vi "HTML Block Diagram Save.vi"(5 "url":string, 7 "title":string="bd.html", 8 "error in":errorcluster, 9 "sub vi loc":T1[](array[typedef]), 10 "sub vi refs":refnum<vi>[](array[refnum]), 11 "base path":path) -> (0 "error out":errorcluster)   [LabVIEW 2014, in "lvprj2html.lvlib"]
uses:
  lvprj2html.lvlib
  <vilib>/Utility/miscctls.llb/LVRectTypeDef.ctl
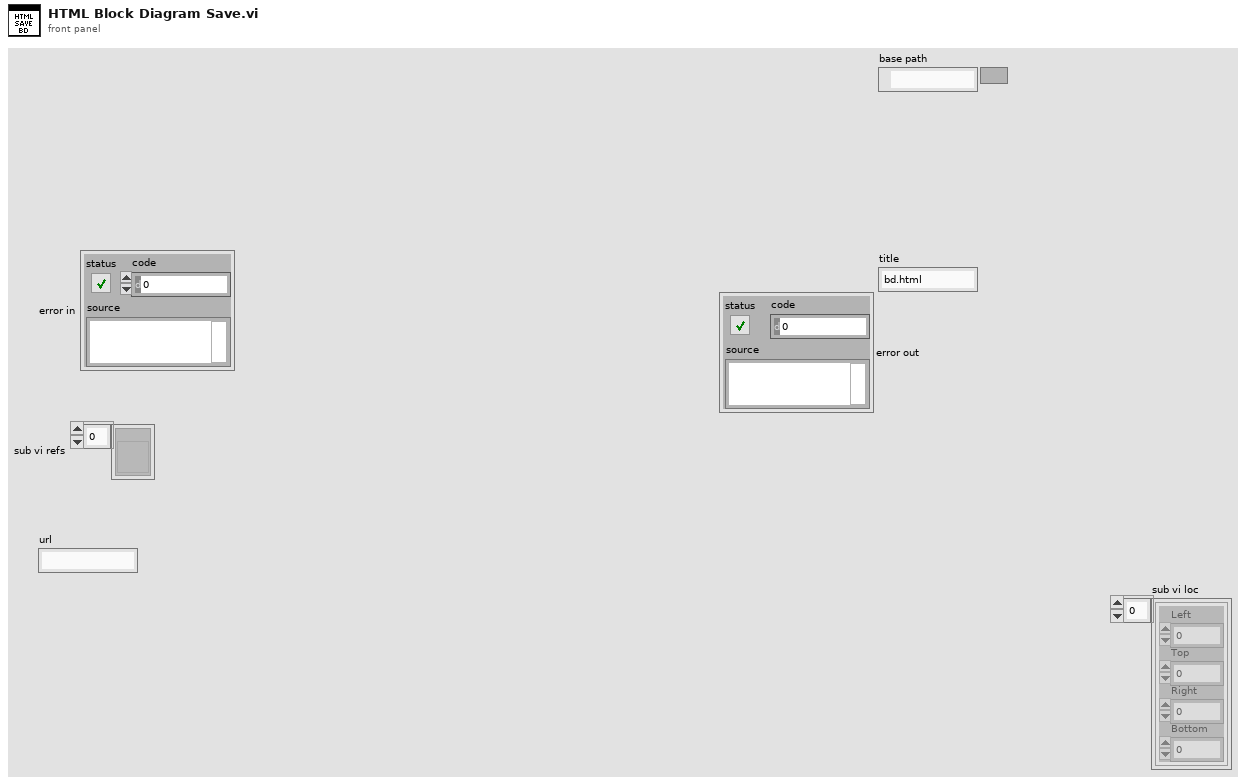
[diagram p1: front panel]
types:
  T1 = typedef "LVRectTypeDef.ctl" = cluster{"Left":i16, "Top":i16, "Right":i16, "Bottom":i16}
  T2 = enum16{"open", "replace", "create", "open or create", "replace or create", "replace or create with confirmation"}
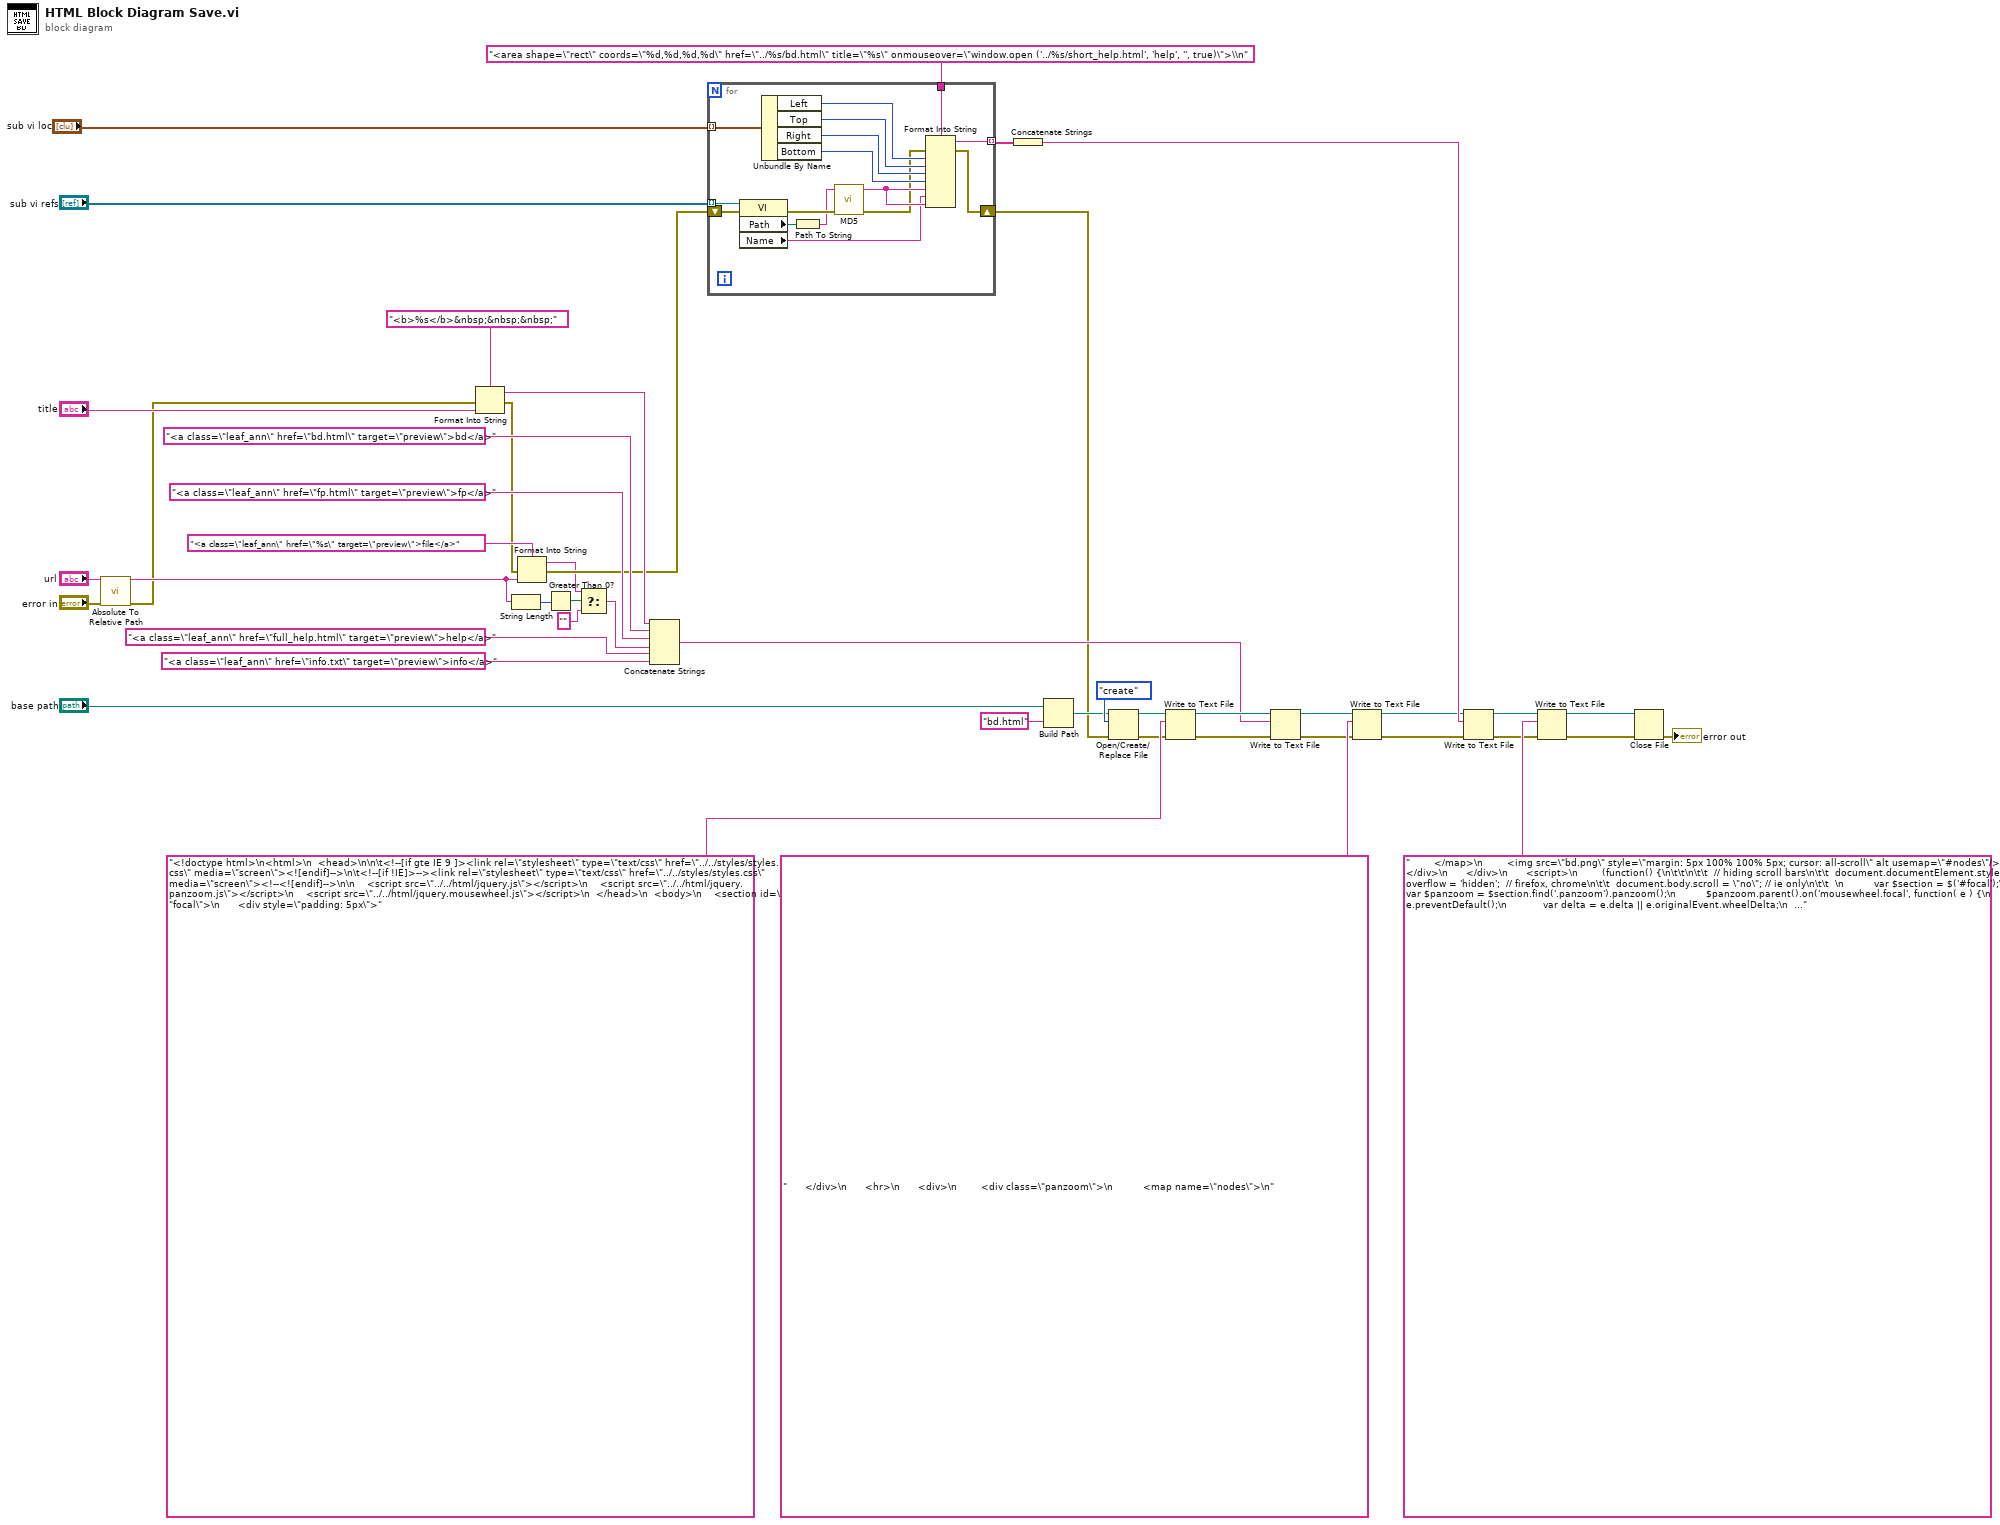
[diagram p0: block diagram]
diagram:
  n1 = call "Absolute To Relative Path.vi"("url in"="url", "error in (no error)"="error in") -> ("url out"=w4:string, "error out"=w3:errorcluster)  [unwired: 12 in]
  n2 = Format Into String(format string="<b>%s</b>&nbsp;&nbsp;&nbsp;", error in=w3, "title") -> (resulting string=w34:string, error out=w13:errorcluster)  [unwired: 1 in]
  n3 = String Length(string=w4) -> (length=w10:i32)
  n4 = Format Into String(format string="<a class=\"leaf_ann\" href=\"%s\" target=\"preview\">file</a>" ("text"), error in=w13, w4) -> (resulting string=w7:string, error out=w12:errorcluster)  [unwired: 1 in]
  n5 = Greater Than 0?(x=w10) -> (x > 0?=w9:bool)
  n6 = Select(t=w7, s=w9, f="") -> (s? t:f=w6:string)
  n7 = Concatenate Strings(w34, "<a class=\"leaf_ann\" href=\"bd.html\" target=\"preview\">bd</a>" ("text"), "<a class=\"leaf_ann\" href=\"fp.html\" target=\"preview\">fp</a>" ("text"), w6, "<a class=\"leaf_ann\" href=\"full_help.html\" target=\"preview\">help</a>" ("text"), "<a class=\"leaf_ann\" href=\"info.txt\" target=\"preview\">info</a>" ("text")) -> (w24:string)
  n8 = for {
    tunnel: "<area shape=\"rect\" coords=\"%d,%d,%d,%d\" href=\"../%s/bd.html\" title=\"%s\" onmouseover=\"window.open ('../%s/short_help.html', 'help', '', true)\">\\n" ("format string") -> [w62]
    tunnel: "sub vi loc" -> [w61] mode=indexing
    tunnel: [w56] -> w39 mode=indexing
    shift-right: [w54] -> w11
    shift-left: w12 -> [w51]
    tunnel: "sub vi refs" -> [w52] mode=indexing
    n9 = property class="VI"(reference=w52, error in=w51) -> (error out=w50:errorcluster, "Path"=w48:path, "Name"=w49:string)  [unwired: 1 out]
    n10 = Unbundle By Name(w61) -> ("Left"=w57:i16, "Top"=w58:i16, "Right"=w59:i16, "Bottom"=w60:i16)
    n11 = Path To String(path=w48) -> (string=w47:string)
    n12 = call "MD5.vi"("error in (no error)"=w50, "Input String"=w47) -> ("error out"=w53:errorcluster, "MD5 message-digest"=w55:string)  [unwired: 8 in]
    n13 = Format Into String(format string=w62, error in=w53, w57, w58, w59, w60, w55, w49, w55) -> (resulting string=w56:string, error out=w54:errorcluster)  [unwired: 1 in]
  }
  n14 = Concatenate Strings(w39) -> (w38:string)
  n15 = Build Path(base path="base path", name or relative path="bd.html") -> (appended path=w44:path)
  n16 = Open/Create/Replace File(file path (use dialog)=w44, error in=w11, operation (0:open)=T2."create") -> (refnum out=w46:refnum<file>, error out=w20:errorcluster)  [unwired: 3 in, 1 out]
  n17 = Write to Text File(file (use dialog)=w46, text="<!doctype html>\n<html>\n  <head>\n\n\t<!--[if gte IE 9 ]><link rel=\"stylesheet\" type=\"text/css\" href=\"../../styles/styles.css\" media=\"screen\"><![endif]-->\n\t<!--[if !IE]>--><link rel=\"stylesheet\" type=\"text/css\" href=\"../../styles/styles.css\" media=\"screen\"><!--<![endif]-->\n\n    <script src=\"../../html/jquery.js\"></script>\n    <script src=\"../../html/jquery.panzoom.js\"></script>\n    <script src=\"../../html/jquery.mousewheel.js\"></script>\n  </head>\n  <body>\n    <section id=\"focal\">\n      <div style=\"padding: 5px\">", error in=w20) -> (refnum out=w27:refnum<file>, error out=w19:errorcluster)  [unwired: 1 in, 1 out]
  n18 = Write to Text File(file (use dialog)=w27, text=w24, error in=w19) -> (refnum out=w26:refnum<file>, error out=w18:errorcluster)  [unwired: 1 in, 1 out]
  n19 = Write to Text File(file (use dialog)=w26, text="      </div>\n      <hr>\n      <div>\n        <div class=\"panzoom\">\n          <map name=\"nodes\">\n", error in=w18) -> (refnum out=w25:refnum<file>, error out=w17:errorcluster)  [unwired: 1 in, 1 out]
  n20 = Write to Text File(file (use dialog)=w25, text=w38, error in=w17) -> (refnum out=w22:refnum<file>, error out=w16:errorcluster)  [unwired: 1 in, 1 out]
  n21 = Write to Text File(file (use dialog)=w22, text="        </map>\n        <img src=\"bd.png\" style=\"margin: 5px 100% 100% 5px; cursor: all-scroll\" alt usemap=\"#nodes\"/>\n        </div>\n      </div>\n      <script>\n        (function() {\n\t\t\n\t\t  // hiding scroll bars\n\t\t  document.documentElement.style.overflow = 'hidden';  // firefox, chrome\n\t\t  document.body.scroll = \"no\"; // ie only\n\t\t  \n          var $section = $('#focal');\n          var $panzoom = $section.find('.panzoom').panzoom();\n          $panzoom.parent().on('mousewheel.focal', function( e ) {\n            e.preventDefault();\n            var delta = e.delta || e.originalEvent.wheelDelta;\n            var zoomOut = delta ? delta < 0 : e.originalEvent.deltaY > 0;\n            $panzoom.panzoom('zoom', zoomOut, {\n              increment: 0.1,\n\t\t\t  minScale: 0.2,\n\t\t\t  maxScale: 1,\n              animate: true,\n              focal: e\n            });\n          });\n        })();\n      </script>\n    </section>\n\n\n  </body>\n</html>", error in=w16) -> (refnum out=w42:refnum<file>, error out=w15:errorcluster)  [unwired: 1 in, 1 out]
  n22 = Close File(refnum=w42, error in=w15) -> (error out=→"error out":errorcluster)  [unwired: 1 out]
